vi "Wait on MovCor window closed.vi"() -> (3 "Timed out waiting":bool)   [LabVIEW 2020]
uses:
  Global Variables/General Globals.vi
panel:
  out "Final Time (s)":dbl format="%#_2f"
  out "Loop iteration":i32
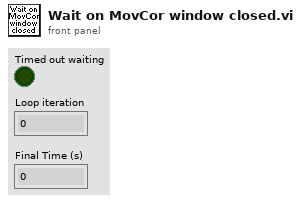
[diagram p1: front panel]
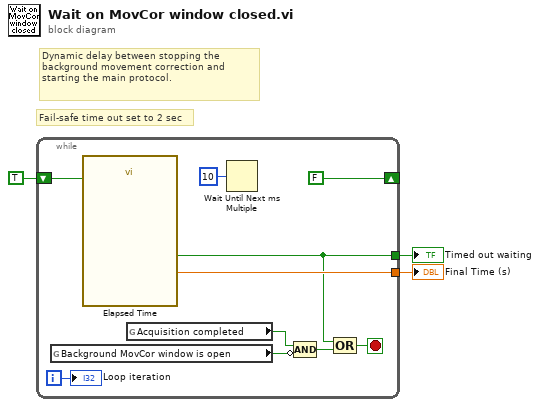
[diagram p0: block diagram]
diagram:
  # "Dynamic delay between stopping the background movement correction and starting the main protocol."
  # "Fail-safe time out set to 2 sec"
  n1 = while {
    shift-right: [FALSE] -> _
    shift-left: TRUE -> [w12]
    tunnel: [w5] -> w3
    tunnel: [w9] -> w2
    i -> [w10]
    stop <- w6 stop-if-true
    n2 = global read "General Globals.vi" "Background MovCor window is open"() -> (w4:bool)
    n3 = call "Elapsed Time"("Reset"=w12) -> ("Elapsed Time (s)"=w9:dbl, "Time has Elapsed"=w5:bool)  [unwired: 11 in, 6 out]
    n4 = global read "General Globals.vi" "Acquisition completed"() -> (w8:bool)
    n5 = Wait Until Next ms Multiple(millisecond multiple=u32 10) -> ()  [unwired: 1 out]
    n6 = Compound Arithmetic op=AND(w8, invert w4) -> (w7:bool)
    n7 = Compound Arithmetic op=OR(w5, w7) -> (w6:bool)
    "Loop iteration" <- w10
  }
  "Timed out waiting" <- w3
  "Final Time (s)" <- w2
